vi "Read TDMS Wavenames.vi"(8 "error in (no error)":errorcluster, 11 "path":path) -> (0 "error out":errorcluster, 2 "Wavenames":string[](array[string]), 3 "file path out":path)   [LabVIEW 2016, in "Data.TDMS.lvclass"]
uses:
  Data.TDMS.lvclass
panel:
  in  "index":i32
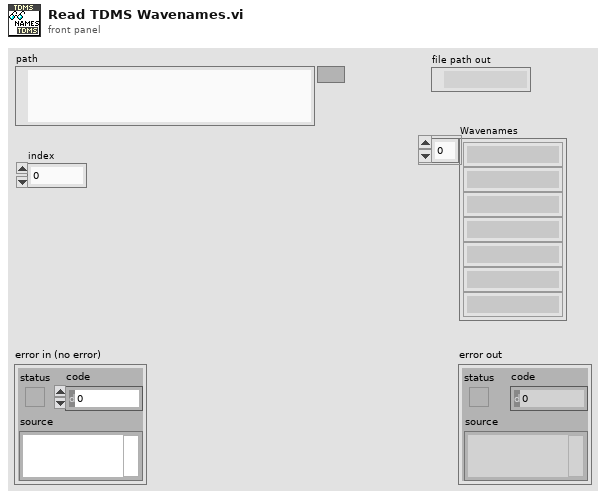
[diagram p1: front panel]
types:
  T1 = enum16{"open", "open or create", "create or replace", "create", "open (read-only)"}
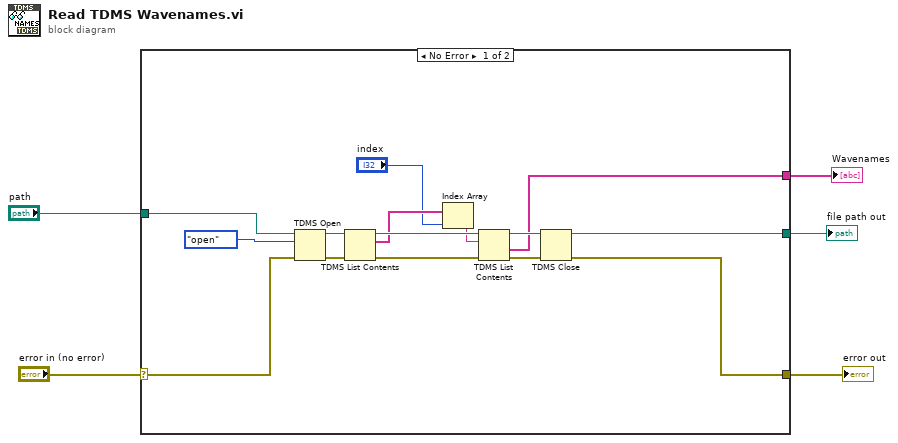
[diagram p0: block diagram]
diagram:
  n1 = case shown="No Error" "error in (no error)" {
    selector: "error in (no error)" -> [w15 w21]
    tunnel: [w19 w21] -> w4
    tunnel: "path" -> [w18 _]
    tunnel: [w14 _] -> w2
    tunnel: [w13 _] -> w1
    frame No Error {
      n2 = TDMS Open(8:w15, 10:T1."open" ("operation (0:open)"), 11:w18) -> (0:w10:errorcluster, 3:w12:refnum<k34>)  [unwired: 4 in]
      n3 = TDMS List Contents(4:w10, 7:w12) -> (0:w9:errorcluster, 2:w8:string[], 3:w11:refnum<k34>)  [unwired: 1 in, 1 out]
      n4 = Index Array(array=w8, index="index") -> (element=w7:string)
      n5 = TDMS List Contents(4:w9, 6:w7, 7:w11) -> (0:w17:errorcluster, 1:w14:string[], 3:w16:refnum<k34>)  [unwired: 1 out]
      n6 = TDMS Close(8:w17, 11:w16) -> (0:w19:errorcluster, 3:w13:path)
    }
    frame Error {
    }
  }
  "error out" <- w4
  "Wavenames" <- w2
  "file path out" <- w1
